vi "PlugIn Joystick.vi"(6 "String Value":string, 10 "Channel":T2, 11 "Menu":T1=enum."set left_rumble") -> ()   [LabVIEW 2019]
uses:
  Joystick Update Ops.ctl
  <vilib>/Rock Robotics/WPI/Joystick/WPI_JoystickDeviceEnum.ctl
panel:
  # "Don't place this VI anywhere\nin your API code. It needs to\nbe a dynamically loaded\nwrapper of the main global"
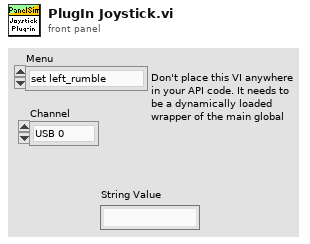
[diagram p1: front panel]
types:
  T1 = typedef "Joystick Update Ops.ctl" = enum16{"set init", "set buttons", "set povs", "set axes", "set left_rumble", "set right_rumble", "set outputs", "get", "delete", "JSON update", "set name", "transmit initial", "reset"}
  T2 = typedef "WPI_JoystickDeviceEnum.ctl" = enum16{"USB 0", "USB 1", "USB 2", "USB 3", "USB 4", "USB 5"}
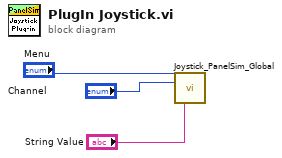
[diagram p0: block diagram]
diagram:
  n1 = call "Joystick_PanelSim_Global.vi"("menu"="Menu", "JoystickDevice"="Channel", "String Value"="String Value") -> ()  [unwired: 11 in, 2 out]
